vi "Waypoint Transfer Status FGV Base.vi"(7 "Method":enum16{"Get", "Set"}(ring), 8 "Error In":errorcluster, 11 "Status In":T1) -> (0 "Error Out":errorcluster, 3 "Waypoint Type Out":T1)   [LabVIEW 2014]
uses:
  Controls/Waypoint Transfer Status.ctl
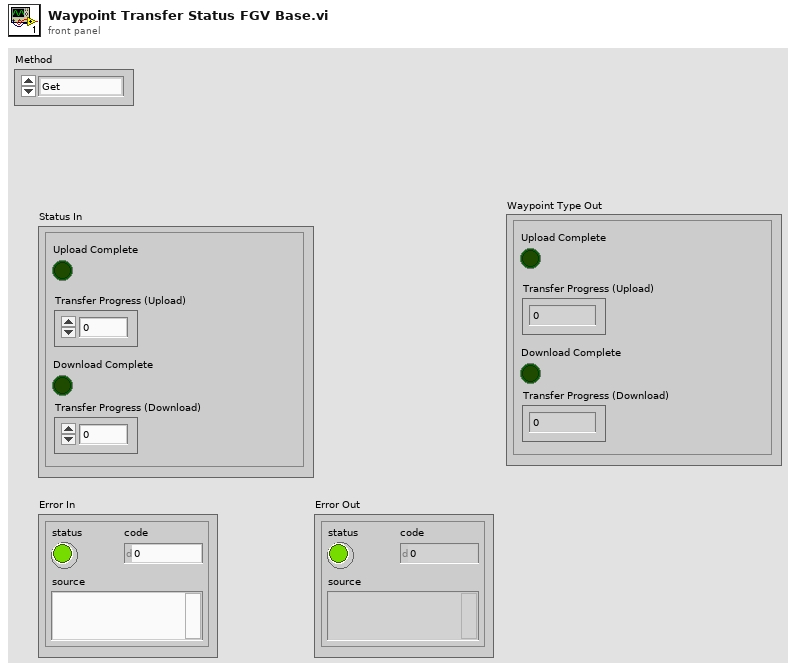
[diagram p1: front panel]
types:
  T1 = typedef "Waypoint Transfer Status.ctl" = cluster{"Upload Complete":bool, "Transfer Progress (Upload)":dbl, "Download Complete":bool, "Transfer Progress (Download)":dbl}
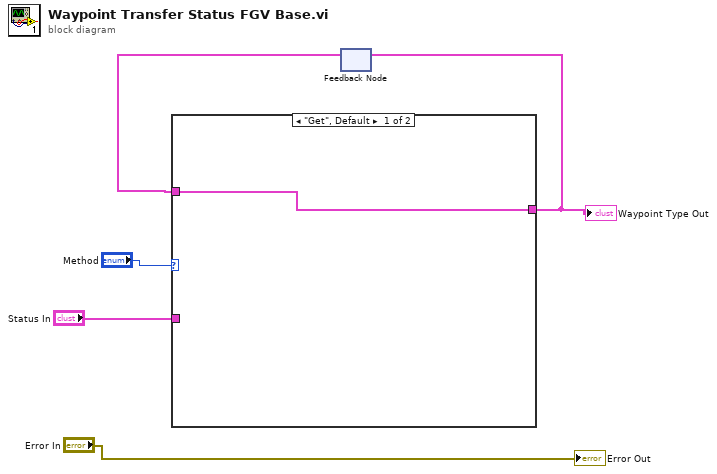
[diagram p0: block diagram]
diagram:
  n1 = feedback #1() -> (w3:T1)  [unwired: 1 in]
  n2 = case shown="\"Get\", Default" "Method" {
    tunnel: "Status In" -> [_ w7]
    tunnel: [w6 w7] -> w2
    tunnel: w3 -> [w6 _]
    frame "Get", Default {
    }
    frame "Set" {
    }
  }
  "Waypoint Type Out" <- w2
  n3 = feedback-in #1(w2) -> ()
  "Error Out" <- "Error In"
